vi "Whether A File or Method.vi"(11 "URI":string) -> (2 "Path(Win)":string, 3 "Type":string)   [LabVIEW 2019, in "HTTP Server.lvlib"]
uses:
  HTTP Server.lvlib
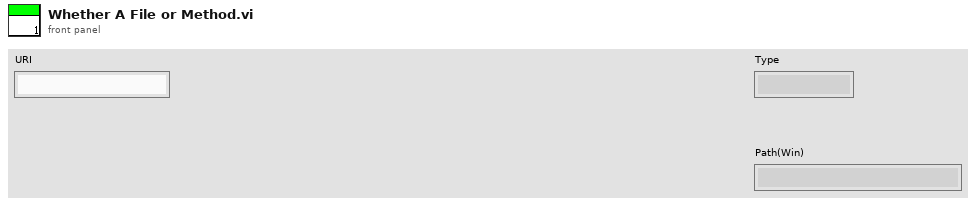
[diagram p1: front panel]
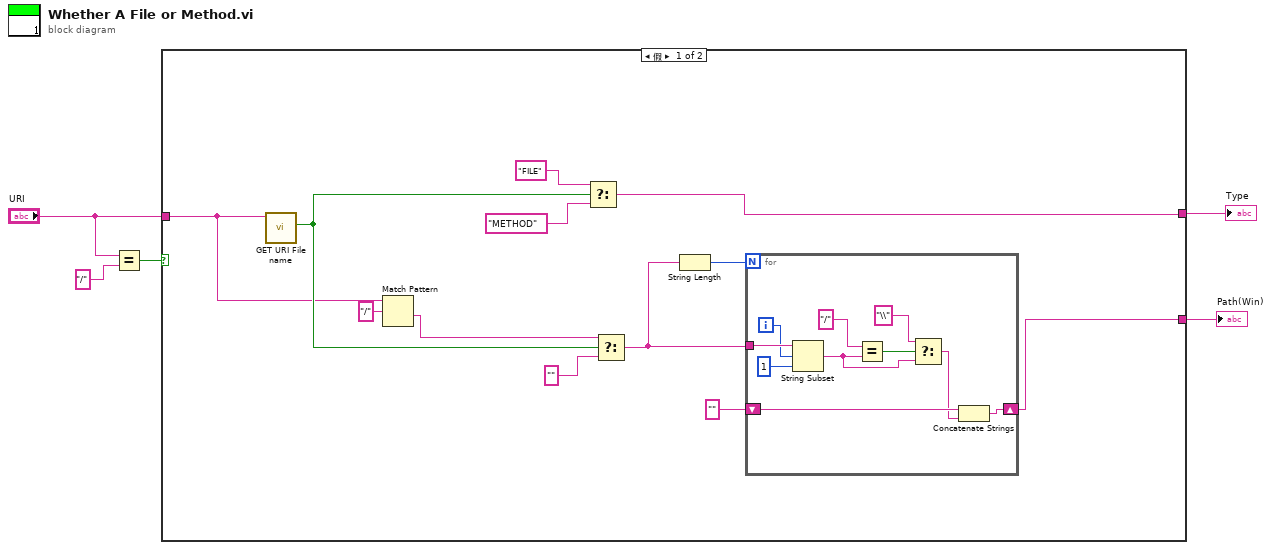
[diagram p0: block diagram]
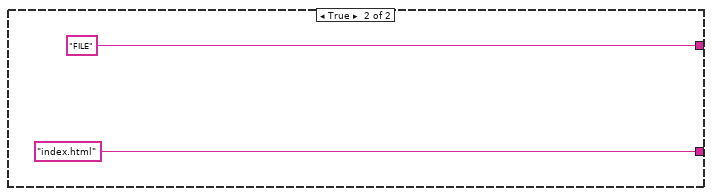
[diagram p2: hidden frame]
diagram:
  n1 = Equal?(x="URI", y="/") -> (x = y?=w4:bool)
  n2 = case shown="假" w4 {
    tunnel: "URI" -> [w12 _]
    tunnel: [w6 "index.html"] -> w1
    tunnel: [w13 "FILE"] -> w2
    frame False {
      n3 = call "GET URI File name.vi"("URI"=w12) -> ("Is File"=w16:bool)  [unwired: 8 in, 2 out]
      n4 = Match Pattern(string=w12, regular expression="/" ("正则表达式")) -> (after substring=w10:string)  [unwired: 1 in, 3 out]
      n5 = Select(t="FILE", s=w16, f="METHOD") -> (s? t:f=w13:string)
      n6 = Select(t=w10, s=w16, f="") -> (s? t:f=w8:string)
      n7 = String Length(string=w8) -> (length=w9:i32)
      n8 = for {
        N: w9 -> [_]
        tunnel: w8 -> [w27]
        shift-right: [w23] -> w6
        shift-left: "" -> [w24]
        i -> [w26]
        n9 = String Subset(string=w27, offset (0)=w26, length (rest)=1 ("长度（剩余）")) -> (substring=w20:string)
        n10 = Equal?(x="/", y=w20) -> (x = y?=w21:bool)
        n11 = Select(t="\\" ("x"), s=w21, f=w20) -> (s? t:f=w18:string)
        n12 = Concatenate Strings(w24, w18) -> (w23:string)
      }
    }
    frame True {
    }
  }
  "Type" <- w2
  "Path(Win)" <- w1
